vi "PAN_WaitObsDone.vi"(8 "error in":errorcluster, 10 "obsID":string, 11 "done queue":refnum<queue>) -> (0 "error out":errorcluster, 2 "response":string)   [LabVIEW 2016]
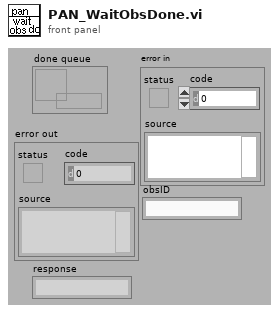
[diagram p1: front panel]
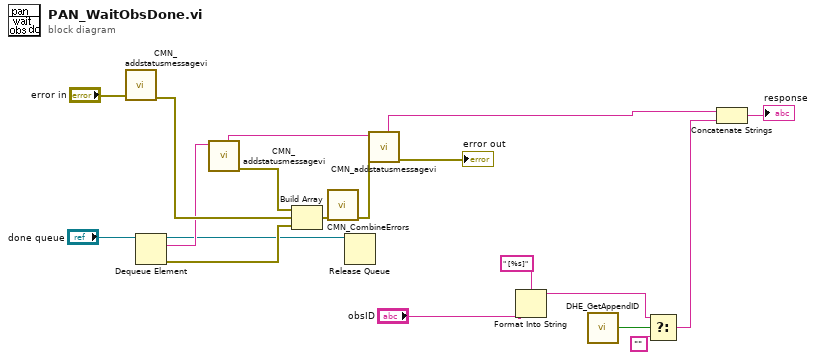
[diagram p0: block diagram]
diagram:
  n1 = call "CMN_addstatusmessagevi.vi"("error in (no error)"="error in") -> ("error out"=w15:errorcluster)  [unwired: 1 in, 9 out]
  n2 = Dequeue Element(queue="done queue") -> (queue out=w10:refnum<queue>, element=w12:string, error out=w11:errorcluster)  [unwired: 1 in, 2 out]
  n3 = call "CMN_addstatusmessagevi.vi"("message  in"=w12) -> ("error out"=w16:errorcluster, "modified message out"=w14:string)  [unwired: 1 in, 8 out]
  n4 = Build Array(w16, w15, w11) -> (w19:errorcluster[])
  n5 = call "CMN_CombineErrors.vi"("Errors"=w19) -> ("error out"=w18:errorcluster)  [unwired: 10 out]
  n6 = Release Queue(queue=w10) -> ()  [unwired: 1 in, 4 out]
  n7 = call "CMN_addstatusmessagevi.vi"("error in (no error)"=w18, "message  in"=w14) -> ("error out"=→"error out":errorcluster, "modified message out"=w17:string)  [unwired: 8 out]
  n8 = Format Into String(format string=" [%s]", "obsID") -> (resulting string=w2:string)  [unwired: 2 in, 1 out]
  n9 = call "DHE_GetAppendID.vi"() -> ("DHE_asyncexp"=w6:bool)  [unwired: 9 out]
  n10 = Select(t=w2, s=w6, f="") -> (s? t:f=w5:string)
  n11 = Concatenate Strings(w17, w5) -> (→"response":string)
